vi "Stop axis.vi"(8 "error in":errorcluster, 10 "Axis to stop":string(combo)="Z") -> (0 "error out":errorcluster)   [LabVIEW 2017]
uses:
  C:/Users/Chip Scope/Desktop/MCM3000- do not delete - critical for LabVIEW stage control/LabVIEW/inc/MCM3000.lvlib
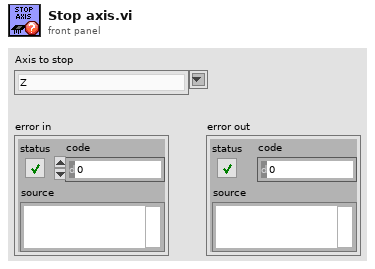
[diagram p1: front panel]
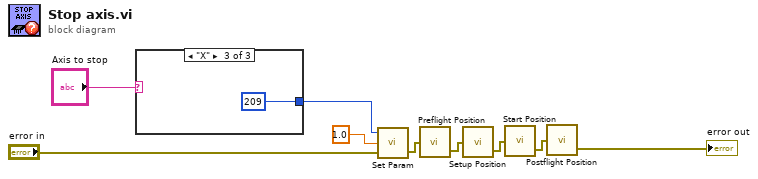
[diagram p0: block diagram]
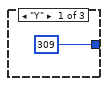
[diagram p2: hidden frame]
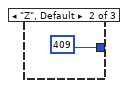
[diagram p3: hidden frame]
diagram:
  n1 = case shown="\"X\"" "Axis to stop" {
    tunnel: [309 ("paramID: PARAM_Z_STOP") 409 ("paramID: PARAM_Z_STOP") 209 ("paramID: PARAM_Z_STOP")] -> w8
    frame "Y" {
    }
    frame "Z", Default {
    }
    frame "X" {
    }
  }
  n2 = call "Set Param.vi"("error in (no error)"="error in", "param"=1.0, "paramID"=w8) -> ("error out"=w7:errorcluster)  [unwired: 1 out]
  n3 = call "Preflight Position.vi"("error in (no error)"=w7) -> ("error out"=w6:errorcluster)  [unwired: 1 out]
  n4 = call "Setup Position.vi"("error in (no error)"=w6) -> ("error out"=w5:errorcluster)  [unwired: 1 out]
  n5 = call "Start Position.vi"("error in (no error)"=w5) -> ("error out"=w4:errorcluster)  [unwired: 1 out]
  n6 = call "Postflight Position.vi"("error in (no error)"=w4) -> ("error out"=→"error out":errorcluster)  [unwired: 1 out]
